vi "response to string.vi"(11 "responses":T1) -> (3 "command string":string)   [LabVIEW 2013, in "module execution process.lvlib"]
uses:
  module execution process.lvlib
  common reponses to network process.ctl
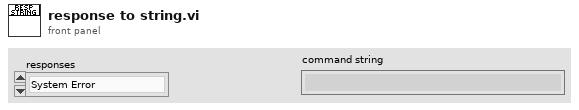
[diagram p1: front panel]
types:
  T1 = typedef "module execution process.lvlib/common reponses to network process.ctl" = enum16{"System Error", "Load Report", "Action Response", "Engine Status"}
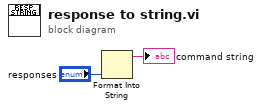
[diagram p0: block diagram]
diagram:
  n1 = Format Into String("responses") -> (resulting string=→"command string":string)  [unwired: 3 in, 1 out]
